vi "Seatingchart.vi"(5 "selected seats before":i32[](array[numeric])) -> (0 "No seat":bool, 1 "selected seats after":i32[](array[numeric]), 2 "seats selected by user":i32[](array[numeric]), 3 "No. of seats choosen":i32, 4 "Cancel":bool)   [LabVIEW 2014]
panel:
  out "No. of seats want to choose":i32
  out "th seat you choose":i32
  out "index":i32
  in  "Seating chart":T1
  in  "stop":bool
  # "1"
  # "2"
  # "3"
  # "4"
  # "5"
  # "6"
  # "A"
  # "A"
  # "B"
  # "B"
  # "C"
  # "C"
  # "D"
  # "D"
  # "E"
  # "E"
  # "F"
  # "F"
  # "G"
  # "G"
  # "H"
  # "H"
  # "1"
  # "2"
  # "3"
  # "4"
  # "5"
  # "6"
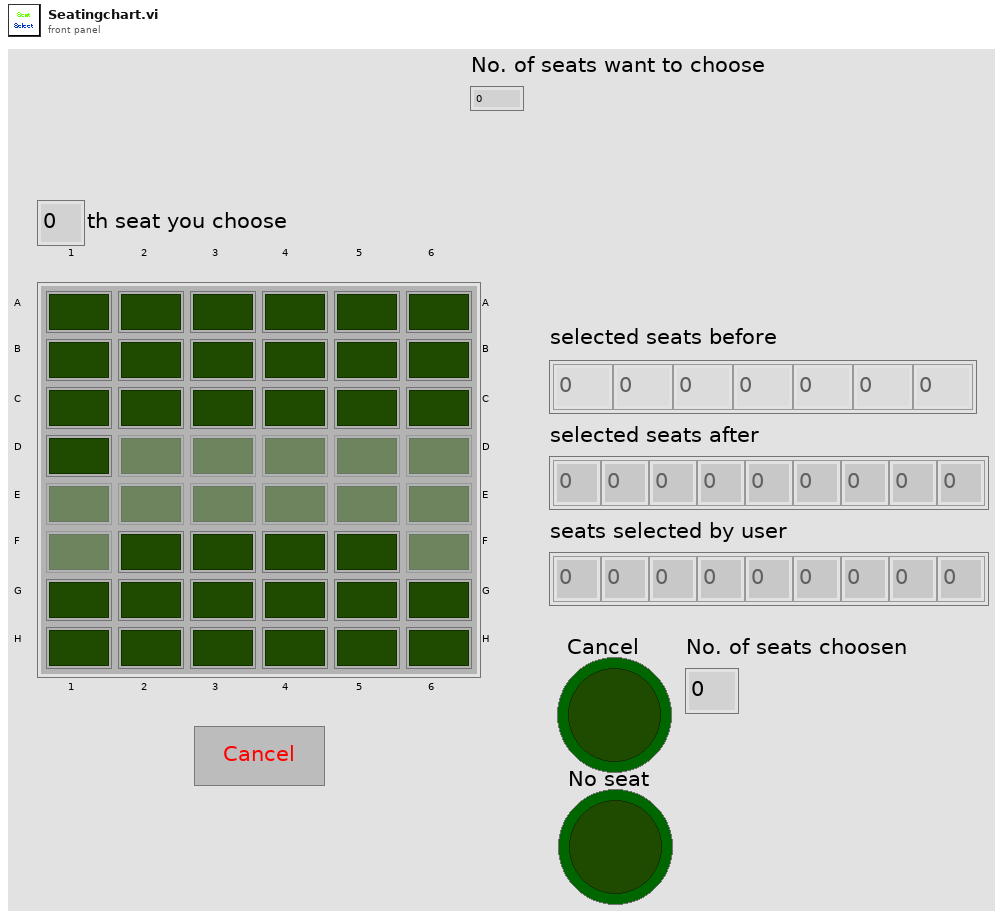
[diagram p1: front panel]
types:
  T1 = cluster{"Boolean":bool, "Boolean 2":bool, "Boolean 3":bool, "Boolean 4":bool, "Boolean 5":bool, "Boolean 6":bool, "Boolean 7":bool, "Boolean 8":bool, "Boolean 9":bool, "Boolean 10":bool, "Boolean 11":bool, "Boolean 12":bool, "Boolean 13":bool, "Boolean 14":bool, "Boolean 15":bool, "Boolean 16":bool, "Boolean 17":bool, "Boolean 18":bool, "Boolean 19":bool, "Boolean 20":bool, "Boolean 21":bool, "Boolean 22":bool, "Boolean 23":bool, "Boolean 24":bool, "Boolean 25":bool, "Boolean 26":bool, "Boolean 27":bool, "Boolean 28":bool, "Boolean 29":bool, "Boolean 30":bool, "Boolean 31":bool, "Boolean 32":bool, "Boolean 33":bool, "Boolean 34":bool, "Boolean 35":bool, "Boolean 36":bool, "Boolean 37":bool, "Boolean 38":bool, "Boolean 39":bool, "Boolean 40":bool, "Boolean 41":bool, "Boolean 42":bool, "Boolean 43":bool, "Boolean 44":bool, "Boolean 45":bool, "Boolean 46":bool, "Boolean 47":bool, "Boolean 48":bool}
  T2 = enum8{"Enabled", "Disabled", "Disabled and Grayed Out"}
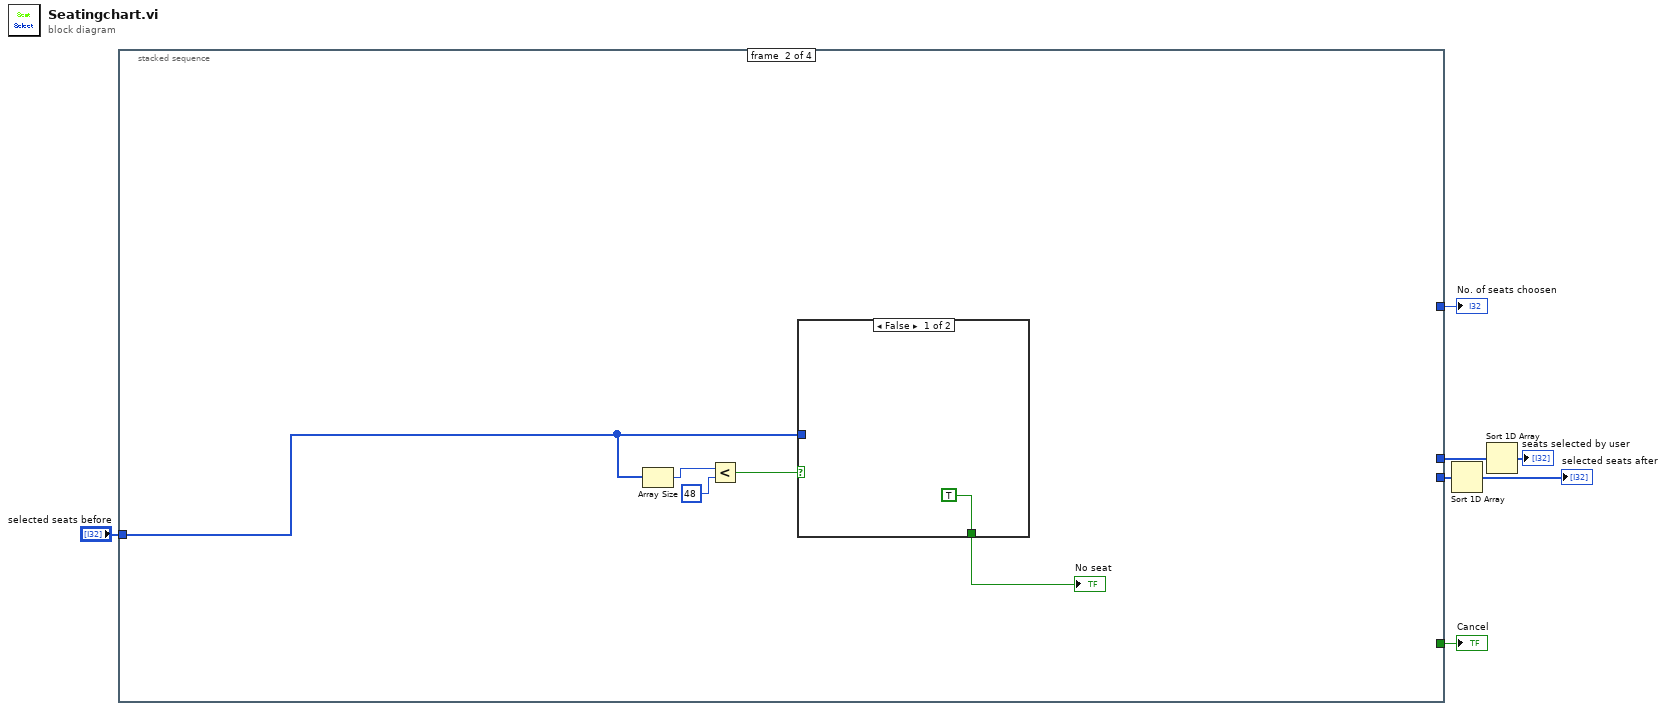
[diagram p0: block diagram]
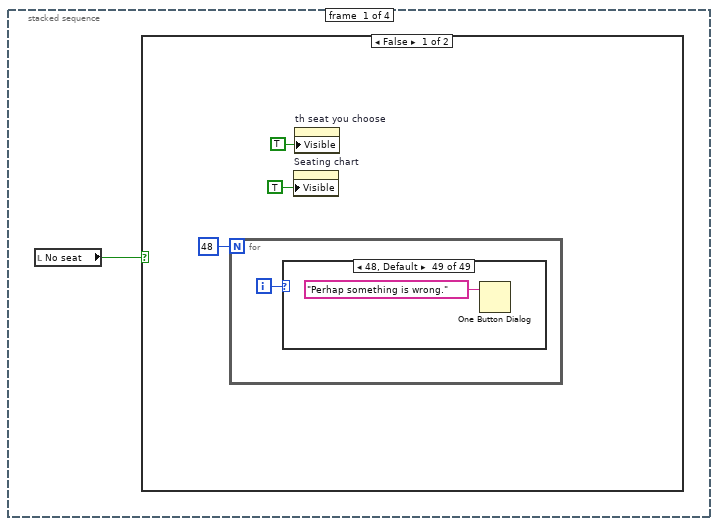
[diagram p2: hidden frame]
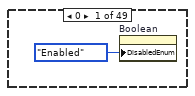
[diagram p3: hidden frame]
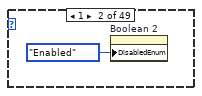
[diagram p4: hidden frame]
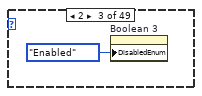
[diagram p5: hidden frame]
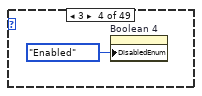
[diagram p6: hidden frame]
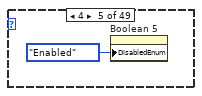
[diagram p7: hidden frame]
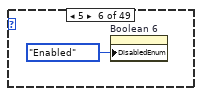
[diagram p8: hidden frame]
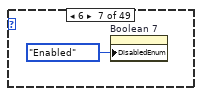
[diagram p9: hidden frame]
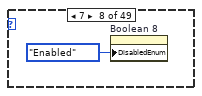
[diagram p10: hidden frame]
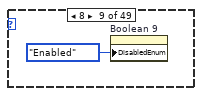
[diagram p11: hidden frame]
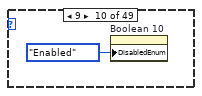
[diagram p12: hidden frame]
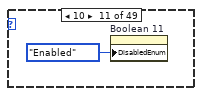
[diagram p13: hidden frame]
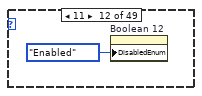
[diagram p14: hidden frame]
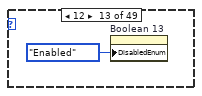
[diagram p15: hidden frame]
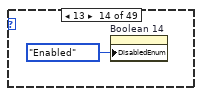
[diagram p16: hidden frame]
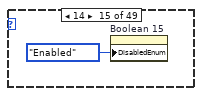
[diagram p17: hidden frame]
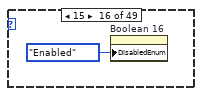
[diagram p18: hidden frame]
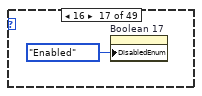
[diagram p19: hidden frame]
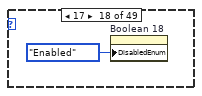
[diagram p20: hidden frame]
diagram:
  n1 = stacked-sequence {
    tunnel: [_ _ _ w130] -> w6
    tunnel: [_ _ _ w128] -> w7
    tunnel: "selected seats before" -> [_ w66 w72 w129]
    tunnel: [_ _ _ w127] -> w4
    tunnel: [_ _ _ w126] -> w3
    frame #0 {
      n2 = local read "No seat"() -> (w8:bool)
      n3 = case shown="False" w8 {
        frame False {
          n4 = for {
            N: 48 -> [_]
            i -> [w12]
            n5 = case shown="48, Default" w12 {
              frame 0 {
                n6 = property on="Boolean" class="Bool"("DisabledEnum"=T2."Enabled" ("Disabled")) -> ()  [unwired: 2 in, 2 out]
              }
              frame 1 {
                n7 = property on="Boolean 2" class="Bool"("DisabledEnum"=T2."Enabled" ("Disabled")) -> ()  [unwired: 2 in, 2 out]
              }
              frame 2 {
                n8 = property on="Boolean 3" class="Bool"("DisabledEnum"=T2."Enabled" ("Disabled")) -> ()  [unwired: 2 in, 2 out]
              }
              frame 3 {
                n9 = property on="Boolean 4" class="Bool"("DisabledEnum"=T2."Enabled" ("Disabled")) -> ()  [unwired: 2 in, 2 out]
              }
              frame 4 {
                n10 = property on="Boolean 5" class="Bool"("DisabledEnum"=T2."Enabled" ("Disabled")) -> ()  [unwired: 2 in, 2 out]
              }
              frame 5 {
                n11 = property on="Boolean 6" class="Bool"("DisabledEnum"=T2."Enabled" ("Disabled")) -> ()  [unwired: 2 in, 2 out]
              }
              frame 6 {
                n12 = property on="Boolean 7" class="Bool"("DisabledEnum"=T2."Enabled" ("Disabled")) -> ()  [unwired: 2 in, 2 out]
              }
              frame 7 {
                n13 = property on="Boolean 8" class="Bool"("DisabledEnum"=T2."Enabled" ("Disabled")) -> ()  [unwired: 2 in, 2 out]
              }
              frame 8 {
                n14 = property on="Boolean 9" class="Bool"("DisabledEnum"=T2."Enabled" ("Disabled")) -> ()  [unwired: 2 in, 2 out]
              }
              frame 9 {
                n15 = property on="Boolean 10" class="Bool"("DisabledEnum"=T2."Enabled" ("Disabled")) -> ()  [unwired: 2 in, 2 out]
              }
              frame 10 {
                n16 = property on="Boolean 11" class="Bool"("DisabledEnum"=T2."Enabled" ("Disabled")) -> ()  [unwired: 2 in, 2 out]
              }
              frame 11 {
                n17 = property on="Boolean 12" class="Bool"("DisabledEnum"=T2."Enabled" ("Disabled")) -> ()  [unwired: 2 in, 2 out]
              }
              frame 12 {
                n18 = property on="Boolean 13" class="Bool"("DisabledEnum"=T2."Enabled" ("Disabled")) -> ()  [unwired: 2 in, 2 out]
              }
              frame 13 {
                n19 = property on="Boolean 14" class="Bool"("DisabledEnum"=T2."Enabled" ("Disabled")) -> ()  [unwired: 2 in, 2 out]
              }
              frame 14 {
                n20 = property on="Boolean 15" class="Bool"("DisabledEnum"=T2."Enabled" ("Disabled")) -> ()  [unwired: 2 in, 2 out]
              }
              frame 15 {
                n21 = property on="Boolean 16" class="Bool"("DisabledEnum"=T2."Enabled" ("Disabled")) -> ()  [unwired: 2 in, 2 out]
              }
              frame 16 {
                n22 = property on="Boolean 17" class="Bool"("DisabledEnum"=T2."Enabled" ("Disabled")) -> ()  [unwired: 2 in, 2 out]
              }
              frame 17 {
                n23 = property on="Boolean 18" class="Bool"("DisabledEnum"=T2."Enabled" ("Disabled")) -> ()  [unwired: 2 in, 2 out]
              }
              frame 18 {
                n24 = property on="Boolean 19" class="Bool"("DisabledEnum"=T2."Enabled" ("Disabled")) -> ()  [unwired: 2 in, 2 out]
              }
              frame 19 {
                n25 = property on="Boolean 20" class="Bool"("DisabledEnum"=T2."Enabled" ("Disabled")) -> ()  [unwired: 2 in, 2 out]
              }
              frame 20 {
                n26 = property on="Boolean 21" class="Bool"("DisabledEnum"=T2."Enabled" ("Disabled")) -> ()  [unwired: 2 in, 2 out]
              }
              frame 21 {
                n27 = property on="Boolean 22" class="Bool"("DisabledEnum"=T2."Enabled" ("Disabled")) -> ()  [unwired: 2 in, 2 out]
              }
              frame 22 {
                n28 = property on="Boolean 23" class="Bool"("DisabledEnum"=T2."Enabled" ("Disabled")) -> ()  [unwired: 2 in, 2 out]
              }
              frame 23 {
                n29 = property on="Boolean 24" class="Bool"("DisabledEnum"=T2."Enabled" ("Disabled")) -> ()  [unwired: 2 in, 2 out]
              }
              frame 24 {
                n30 = property on="Boolean 25" class="Bool"("DisabledEnum"=T2."Enabled" ("Disabled")) -> ()  [unwired: 2 in, 2 out]
              }
              frame 25 {
                n31 = property on="Boolean 26" class="Bool"("DisabledEnum"=T2."Enabled" ("Disabled")) -> ()  [unwired: 2 in, 2 out]
              }
              frame 26 {
                n32 = property on="Boolean 27" class="Bool"("DisabledEnum"=T2."Enabled" ("Disabled")) -> ()  [unwired: 2 in, 2 out]
              }
              frame 27 {
                n33 = property on="Boolean 28" class="Bool"("DisabledEnum"=T2."Enabled" ("Disabled")) -> ()  [unwired: 2 in, 2 out]
              }
              frame 28 {
                n34 = property on="Boolean 29" class="Bool"("DisabledEnum"=T2."Enabled" ("Disabled")) -> ()  [unwired: 2 in, 2 out]
              }
              frame 29 {
                n35 = property on="Boolean 30" class="Bool"("DisabledEnum"=T2."Enabled" ("Disabled")) -> ()  [unwired: 2 in, 2 out]
              }
              frame 30 {
                n36 = property on="Boolean 31" class="Bool"("DisabledEnum"=T2."Enabled" ("Disabled")) -> ()  [unwired: 2 in, 2 out]
              }
              frame 31 {
                n37 = property on="Boolean 32" class="Bool"("DisabledEnum"=T2."Enabled" ("Disabled")) -> ()  [unwired: 2 in, 2 out]
              }
              frame 32 {
                n38 = property on="Boolean 33" class="Bool"("DisabledEnum"=T2."Enabled" ("Disabled")) -> ()  [unwired: 2 in, 2 out]
              }
              frame 33 {
                n39 = property on="Boolean 34" class="Bool"("DisabledEnum"=T2."Enabled" ("Disabled")) -> ()  [unwired: 2 in, 2 out]
              }
              frame 34 {
                n40 = property on="Boolean 35" class="Bool"("DisabledEnum"=T2."Enabled" ("Disabled")) -> ()  [unwired: 2 in, 2 out]
              }
              frame 35 {
                n41 = property on="Boolean 36" class="Bool"("DisabledEnum"=T2."Enabled" ("Disabled")) -> ()  [unwired: 2 in, 2 out]
              }
              frame 36 {
                n42 = property on="Boolean 37" class="Bool"("DisabledEnum"=T2."Enabled" ("Disabled")) -> ()  [unwired: 2 in, 2 out]
              }
              frame 37 {
                n43 = property on="Boolean 38" class="Bool"("DisabledEnum"=T2."Enabled" ("Disabled")) -> ()  [unwired: 2 in, 2 out]
              }
              frame 38 {
                n44 = property on="Boolean 39" class="Bool"("DisabledEnum"=T2."Enabled" ("Disabled")) -> ()  [unwired: 2 in, 2 out]
              }
              frame 39 {
                n45 = property on="Boolean 40" class="Bool"("DisabledEnum"=T2."Enabled" ("Disabled")) -> ()  [unwired: 2 in, 2 out]
              }
              frame 40 {
                n46 = property on="Boolean 41" class="Bool"("DisabledEnum"=T2."Enabled" ("Disabled")) -> ()  [unwired: 2 in, 2 out]
              }
              frame 41 {
                n47 = property on="Boolean 42" class="Bool"("DisabledEnum"=T2."Enabled" ("Disabled")) -> ()  [unwired: 2 in, 2 out]
              }
              frame 42 {
                n48 = property on="Boolean 43" class="Bool"("DisabledEnum"=T2."Enabled" ("Disabled")) -> ()  [unwired: 2 in, 2 out]
              }
              frame 43 {
                n49 = property on="Boolean 44" class="Bool"("DisabledEnum"=T2."Enabled" ("Disabled")) -> ()  [unwired: 2 in, 2 out]
              }
              frame 44 {
                n50 = property on="Boolean 45" class="Bool"("DisabledEnum"=T2."Enabled" ("Disabled")) -> ()  [unwired: 2 in, 2 out]
              }
              frame 45 {
                n51 = property on="Boolean 46" class="Bool"("DisabledEnum"=T2."Enabled" ("Disabled")) -> ()  [unwired: 2 in, 2 out]
              }
              frame 46 {
                n52 = property on="Boolean 47" class="Bool"("DisabledEnum"=T2."Enabled" ("Disabled")) -> ()  [unwired: 2 in, 2 out]
              }
              frame 47 {
                n53 = property on="Boolean 48" class="Bool"("DisabledEnum"=T2."Enabled" ("Disabled")) -> ()  [unwired: 2 in, 2 out]
              }
              frame 48, Default {
                n54 = One Button Dialog(message="Perhap something is wrong.") -> ()  [unwired: 1 in, 1 out]
              }
            }
          }
          n55 = property on="Seating chart" class="Clust"("Visible"=TRUE) -> ()  [unwired: 2 in, 2 out]
          n56 = property on="th seat you choose" class="DigNum (strict)"("Visible"=TRUE) -> ()  [unwired: 2 in, 2 out]
        }
        frame True {
        }
      }
    }
    frame #1 {
      n57 = Array Size(array=w66) -> (size(s)=w62:i32)
      n58 = Less?(x=w62, y=48 ("x")) -> (x < y?=w65:bool)
      n59 = case shown="False" w65 {
        tunnel: w66 -> [_ w70]
        tunnel: [TRUE FALSE] -> w64
        frame False {
        }
        frame True {
          n60 = call "how_many_seats.vi"("selected seats before"=w70) -> ("How many seats do \nyou want to choose?\n(O)"=→"No. of seats want to choose":i32)
        }
      }
      "No seat" <- w64
    }
    frame #2 {
      n61 = local read "No seat"() -> (w71:bool)
      n62 = case shown="False" w71 {
        tunnel: w72 -> [w73 _]
        frame False {
          n63 = Array Size(array=w73) -> (size(s)=w74:i32)
          n64 = for {
            N: w74 -> [_]
            tunnel: w73 -> [w75] mode=indexing
            n65 = case shown="48, Default" w75 {
              frame 0 {
                n66 = property on="Boolean" class="Bool"("DisabledEnum"=T2."Disabled and Grayed Out" ("Disabled")) -> ()  [unwired: 2 in, 2 out]
              }
              frame 1 {
                n67 = property on="Boolean 2" class="Bool"("DisabledEnum"=T2."Disabled and Grayed Out" ("Disabled")) -> ()  [unwired: 2 in, 2 out]
              }
              frame 2 {
                n68 = property on="Boolean 3" class="Bool"("DisabledEnum"=T2."Disabled and Grayed Out" ("Disabled")) -> ()  [unwired: 2 in, 2 out]
              }
              frame 3 {
                n69 = property on="Boolean 4" class="Bool"("DisabledEnum"=T2."Disabled and Grayed Out" ("Disabled")) -> ()  [unwired: 2 in, 2 out]
              }
              frame 4 {
                n70 = property on="Boolean 5" class="Bool"("DisabledEnum"=T2."Disabled and Grayed Out" ("Disabled")) -> ()  [unwired: 2 in, 2 out]
              }
              frame 5 {
                n71 = property on="Boolean 6" class="Bool"("DisabledEnum"=T2."Disabled and Grayed Out" ("Disabled")) -> ()  [unwired: 2 in, 2 out]
              }
              frame 6 {
                n72 = property on="Boolean 7" class="Bool"("DisabledEnum"=T2."Disabled and Grayed Out" ("Disabled")) -> ()  [unwired: 2 in, 2 out]
              }
              frame 7 {
                n73 = property on="Boolean 8" class="Bool"("DisabledEnum"=T2."Disabled and Grayed Out" ("Disabled")) -> ()  [unwired: 2 in, 2 out]
              }
              frame 8 {
                n74 = property on="Boolean 9" class="Bool"("DisabledEnum"=T2."Disabled and Grayed Out" ("Disabled")) -> ()  [unwired: 2 in, 2 out]
              }
              frame 9 {
                n75 = property on="Boolean 10" class="Bool"("DisabledEnum"=T2."Disabled and Grayed Out" ("Disabled")) -> ()  [unwired: 2 in, 2 out]
              }
              frame 10 {
                n76 = property on="Boolean 11" class="Bool"("DisabledEnum"=T2."Disabled and Grayed Out" ("Disabled")) -> ()  [unwired: 2 in, 2 out]
              }
              frame 11 {
                n77 = property on="Boolean 12" class="Bool"("DisabledEnum"=T2."Disabled and Grayed Out" ("Disabled")) -> ()  [unwired: 2 in, 2 out]
              }
              frame 12 {
                n78 = property on="Boolean 13" class="Bool"("DisabledEnum"=T2."Disabled and Grayed Out" ("Disabled")) -> ()  [unwired: 2 in, 2 out]
              }
              frame 13 {
                n79 = property on="Boolean 14" class="Bool"("DisabledEnum"=T2."Disabled and Grayed Out" ("Disabled")) -> ()  [unwired: 2 in, 2 out]
              }
              frame 14 {
                n80 = property on="Boolean 15" class="Bool"("DisabledEnum"=T2."Disabled and Grayed Out" ("Disabled")) -> ()  [unwired: 2 in, 2 out]
              }
              frame 15 {
                n81 = property on="Boolean 16" class="Bool"("DisabledEnum"=T2."Disabled and Grayed Out" ("Disabled")) -> ()  [unwired: 2 in, 2 out]
              }
              frame 16 {
                n82 = property on="Boolean 17" class="Bool"("DisabledEnum"=T2."Disabled and Grayed Out" ("Disabled")) -> ()  [unwired: 2 in, 2 out]
              }
              frame 17 {
                n83 = property on="Boolean 18" class="Bool"("DisabledEnum"=T2."Disabled and Grayed Out" ("Disabled")) -> ()  [unwired: 2 in, 2 out]
              }
              frame 18 {
                n84 = property on="Boolean 19" class="Bool"("DisabledEnum"=T2."Disabled and Grayed Out" ("Disabled")) -> ()  [unwired: 2 in, 2 out]
              }
              frame 19 {
                n85 = property on="Boolean 20" class="Bool"("DisabledEnum"=T2."Disabled and Grayed Out" ("Disabled")) -> ()  [unwired: 2 in, 2 out]
              }
              frame 20 {
                n86 = property on="Boolean 21" class="Bool"("DisabledEnum"=T2."Disabled and Grayed Out" ("Disabled")) -> ()  [unwired: 2 in, 2 out]
              }
              frame 21 {
                n87 = property on="Boolean 22" class="Bool"("DisabledEnum"=T2."Disabled and Grayed Out" ("Disabled")) -> ()  [unwired: 2 in, 2 out]
              }
              frame 22 {
                n88 = property on="Boolean 23" class="Bool"("DisabledEnum"=T2."Disabled and Grayed Out" ("Disabled")) -> ()  [unwired: 2 in, 2 out]
              }
              frame 23 {
                n89 = property on="Boolean 24" class="Bool"("DisabledEnum"=T2."Disabled and Grayed Out" ("Disabled")) -> ()  [unwired: 2 in, 2 out]
              }
              frame 24 {
                n90 = property on="Boolean 25" class="Bool"("DisabledEnum"=T2."Disabled and Grayed Out" ("Disabled")) -> ()  [unwired: 2 in, 2 out]
              }
              frame 25 {
                n91 = property on="Boolean 26" class="Bool"("DisabledEnum"=T2."Disabled and Grayed Out" ("Disabled")) -> ()  [unwired: 2 in, 2 out]
              }
              frame 26 {
                n92 = property on="Boolean 27" class="Bool"("DisabledEnum"=T2."Disabled and Grayed Out" ("Disabled")) -> ()  [unwired: 2 in, 2 out]
              }
              frame 27 {
                n93 = property on="Boolean 28" class="Bool"("DisabledEnum"=T2."Disabled and Grayed Out" ("Disabled")) -> ()  [unwired: 2 in, 2 out]
              }
              frame 28 {
                n94 = property on="Boolean 29" class="Bool"("DisabledEnum"=T2."Disabled and Grayed Out" ("Disabled")) -> ()  [unwired: 2 in, 2 out]
              }
              frame 29 {
                n95 = property on="Boolean 30" class="Bool"("DisabledEnum"=T2."Disabled and Grayed Out" ("Disabled")) -> ()  [unwired: 2 in, 2 out]
              }
              frame 30 {
                n96 = property on="Boolean 31" class="Bool"("DisabledEnum"=T2."Disabled and Grayed Out" ("Disabled")) -> ()  [unwired: 2 in, 2 out]
              }
              frame 31 {
                n97 = property on="Boolean 32" class="Bool"("DisabledEnum"=T2."Disabled and Grayed Out" ("Disabled")) -> ()  [unwired: 2 in, 2 out]
              }
              frame 32 {
                n98 = property on="Boolean 33" class="Bool"("DisabledEnum"=T2."Disabled and Grayed Out" ("Disabled")) -> ()  [unwired: 2 in, 2 out]
              }
              frame 33 {
                n99 = property on="Boolean 34" class="Bool"("DisabledEnum"=T2."Disabled and Grayed Out" ("Disabled")) -> ()  [unwired: 2 in, 2 out]
              }
              frame 34 {
                n100 = property on="Boolean 35" class="Bool"("DisabledEnum"=T2."Disabled and Grayed Out" ("Disabled")) -> ()  [unwired: 2 in, 2 out]
              }
              frame 35 {
                n101 = property on="Boolean 36" class="Bool"("DisabledEnum"=T2."Disabled and Grayed Out" ("Disabled")) -> ()  [unwired: 2 in, 2 out]
              }
              frame 36 {
                n102 = property on="Boolean 37" class="Bool"("DisabledEnum"=T2."Disabled and Grayed Out" ("Disabled")) -> ()  [unwired: 2 in, 2 out]
              }
              frame 37 {
                n103 = property on="Boolean 38" class="Bool"("DisabledEnum"=T2."Disabled and Grayed Out" ("Disabled")) -> ()  [unwired: 2 in, 2 out]
              }
              frame 38 {
                n104 = property on="Boolean 39" class="Bool"("DisabledEnum"=T2."Disabled and Grayed Out" ("Disabled")) -> ()  [unwired: 2 in, 2 out]
              }
              frame 39 {
                n105 = property on="Boolean 40" class="Bool"("DisabledEnum"=T2."Disabled and Grayed Out" ("Disabled")) -> ()  [unwired: 2 in, 2 out]
              }
              frame 40 {
                n106 = property on="Boolean 41" class="Bool"("DisabledEnum"=T2."Disabled and Grayed Out" ("Disabled")) -> ()  [unwired: 2 in, 2 out]
              }
              frame 41 {
                n107 = property on="Boolean 42" class="Bool"("DisabledEnum"=T2."Disabled and Grayed Out" ("Disabled")) -> ()  [unwired: 2 in, 2 out]
              }
              frame 42 {
                n108 = property on="Boolean 43" class="Bool"("DisabledEnum"=T2."Disabled and Grayed Out" ("Disabled")) -> ()  [unwired: 2 in, 2 out]
              }
              frame 43 {
                n109 = property on="Boolean 44" class="Bool"("DisabledEnum"=T2."Disabled and Grayed Out" ("Disabled")) -> ()  [unwired: 2 in, 2 out]
              }
              frame 44 {
                n110 = property on="Boolean 45" class="Bool"("DisabledEnum"=T2."Disabled and Grayed Out" ("Disabled")) -> ()  [unwired: 2 in, 2 out]
              }
              frame 45 {
                n111 = property on="Boolean 46" class="Bool"("DisabledEnum"=T2."Disabled and Grayed Out" ("Disabled")) -> ()  [unwired: 2 in, 2 out]
              }
              frame 46 {
                n112 = property on="Boolean 47" class="Bool"("DisabledEnum"=T2."Disabled and Grayed Out" ("Disabled")) -> ()  [unwired: 2 in, 2 out]
              }
              frame 47 {
                n113 = property on="Boolean 48" class="Bool"("DisabledEnum"=T2."Disabled and Grayed Out" ("Disabled")) -> ()  [unwired: 2 in, 2 out]
              }
              frame 48, Default {
                n114 = One Button Dialog(message="Perhap something is wrong.") -> ()  [unwired: 1 in, 1 out]
              }
            }
          }
        }
        frame True {
        }
      }
    }
    frame #3 {
      n115 = local read "No seat"() -> (w125:bool)
      n116 = case shown="True" w125 {
        tunnel: [w138 w836] -> w130
        tunnel: w129 -> [w136 _]
        tunnel: [w135 w836] -> w128
        tunnel: [w134 FALSE ("stop")] -> w127
        tunnel: [w132 0 ("No. of seats want to choose")] -> w126
        frame False {
          n117 = local read "No. of seats want to choose"() -> (w133:i32)
          n118 = while {
            shift-right: [w151] -> _
            shift-left: w133 -> [w150]
            shift-right: [w156] -> w137
            shift-left: i32[] [] ("Array") -> [w157]
            tunnel: ["stop"] -> w134
            tunnel: w133 -> [w147]
            tunnel: [w147] -> w131
            stop <- w154 stop-if-true
            n119 = Cluster To Array(cluster="Seating chart") -> (array=w158:bool[])
            n120 = Search 1D Array(1D array=w158, element=TRUE) -> (index of element=w155:i32)  [unwired: 1 in]
            "index" <- w155
            n121 = case shown="47" w155 {
              selector: w155 -> [w161 w175 w189 w203 w217 w231 w245 w259 w273 w287 w301 w315 w329 w343 w357 w371 w385 w399 w413 w427 w441 w455 w469 w483 w497 w511 w525 w539 w553 w567 w581 w595 w609 w623 w637 w651 w665 w679 w693 w707 w721 w735 w749 w763 w777 w791 w805 w819 _]
              tunnel: w150 -> [w165 w179 w193 w207 w221 w235 w249 w263 w277 w291 w305 w319 w333 w347 w361 w375 w389 w403 w417 w431 w445 w459 w473 w487 w501 w515 w529 w543 w557 w571 w585 w599 w613 w627 w641 w655 w669 w683 w697 w711 w725 w739 w753 w767 w781 w795 w809 w823 w834]
              tunnel: [w164 w178 w192 w206 w220 w234 w248 w262 w276 w290 w304 w318 w332 w346 w360 w374 w388 w402 w416 w430 w444 w458 w472 w486 w500 w514 w528 w542 w556 w570 w584 w598 w612 w626 w640 w654 w668 w682 w696 w710 w724 w738 w752 w766 w780 w794 w808 w822 w834] -> w151
              tunnel: w157 -> [w163 w177 w191 w205 w219 w233 w247 w261 w275 w289 w303 w317 w331 w345 w359 w373 w387 w401 w415 w429 w443 w457 w471 w485 w499 w513 w527 w541 w555 w569 w583 w597 w611 w625 w639 w653 w667 w681 w695 w709 w723 w737 w751 w765 w779 w793 w807 w821 w833]
              tunnel: [w162 w176 w190 w204 w218 w232 w246 w260 w274 w288 w302 w316 w330 w344 w358 w372 w386 w400 w414 w428 w442 w456 w470 w484 w498 w512 w526 w540 w554 w568 w582 w596 w610 w624 w638 w652 w666 w680 w694 w708 w722 w736 w750 w764 w778 w792 w806 w820 w833] -> w156
              frame 0 {
                n122 = call "select_seat_comfirm.vi"("choose index"=w161) -> ("Boolean"=w166:bool)
                n123 = case shown="True" w166 {
                  tunnel: w165 -> [w168 w173]
                  tunnel: [w168 w172] -> w164
                  tunnel: w163 -> [w167 w171]
                  tunnel: [w167 w169] -> w162
                  tunnel: w161 -> [_ w170]
                  frame False {
                  }
                  frame True {
                    n124 = Build Array (concatenate)(w171, w170) -> (w169:i32[])
                    n125 = Decrement(x=w173) -> (x-1=w172:i32)
                    n126 = property on="Boolean" class="Bool"("DisabledEnum"=T2."Disabled and Grayed Out" ("Disabled")) -> ()  [unwired: 2 in, 2 out]
                  }
                }
              }
              frame 1 {
                n127 = call "select_seat_comfirm.vi"("choose index"=w175) -> ("Boolean"=w180:bool)
                n128 = case shown="True" w180 {
                  tunnel: w179 -> [w182 w188]
                  tunnel: [w182 w187] -> w178
                  tunnel: w177 -> [w181 w186]
                  tunnel: [w181 w184] -> w176
                  tunnel: w175 -> [_ w185]
                  frame False {
                  }
                  frame True {
                    n129 = Build Array (concatenate)(w186, w185) -> (w184:i32[])
                    n130 = Decrement(x=w188) -> (x-1=w187:i32)
                    n131 = property on="Boolean 2" class="Bool"("DisabledEnum"=T2."Disabled and Grayed Out" ("Disabled")) -> ()  [unwired: 2 in, 2 out]
                  }
                }
              }
              frame 2 {
                n132 = call "select_seat_comfirm.vi"("choose index"=w189) -> ("Boolean"=w194:bool)
                n133 = case shown="True" w194 {
                  tunnel: w193 -> [w196 w202]
                  tunnel: [w196 w201] -> w192
                  tunnel: w191 -> [w195 w200]
                  tunnel: [w195 w198] -> w190
                  tunnel: w189 -> [_ w199]
                  frame False {
                  }
                  frame True {
                    n134 = Build Array (concatenate)(w200, w199) -> (w198:i32[])
                    n135 = Decrement(x=w202) -> (x-1=w201:i32)
                    n136 = property on="Boolean 3" class="Bool"("DisabledEnum"=T2."Disabled and Grayed Out" ("Disabled")) -> ()  [unwired: 2 in, 2 out]
                  }
                }
              }
              frame 3 {
                n137 = call "select_seat_comfirm.vi"("choose index"=w203) -> ("Boolean"=w208:bool)
                n138 = case shown="True" w208 {
                  tunnel: w207 -> [w210 w216]
                  tunnel: [w210 w215] -> w206
                  tunnel: w205 -> [w209 w214]
                  tunnel: [w209 w212] -> w204
                  tunnel: w203 -> [_ w213]
                  frame False {
                  }
                  frame True {
                    n139 = Build Array (concatenate)(w214, w213) -> (w212:i32[])
                    n140 = Decrement(x=w216) -> (x-1=w215:i32)
                    n141 = property on="Boolean 4" class="Bool"("DisabledEnum"=T2."Disabled and Grayed Out" ("Disabled")) -> ()  [unwired: 2 in, 2 out]
                  }
                }
              }
              frame 4 {
                n142 = call "select_seat_comfirm.vi"("choose index"=w217) -> ("Boolean"=w222:bool)
                n143 = case shown="True" w222 {
                  tunnel: w221 -> [w224 w230]
                  tunnel: [w224 w229] -> w220
                  tunnel: w219 -> [w223 w228]
                  tunnel: [w223 w226] -> w218
                  tunnel: w217 -> [_ w227]
                  frame False {
                  }
                  frame True {
                    n144 = Build Array (concatenate)(w228, w227) -> (w226:i32[])
                    n145 = Decrement(x=w230) -> (x-1=w229:i32)
                    n146 = property on="Boolean 5" class="Bool"("DisabledEnum"=T2."Disabled and Grayed Out" ("Disabled")) -> ()  [unwired: 2 in, 2 out]
                  }
                }
              }
              frame 5 {
                n147 = call "select_seat_comfirm.vi"("choose index"=w231) -> ("Boolean"=w236:bool)
                n148 = case shown="True" w236 {
                  tunnel: w235 -> [w238 w244]
                  tunnel: [w238 w243] -> w234
                  tunnel: w233 -> [w237 w242]
                  tunnel: [w237 w240] -> w232
                  tunnel: w231 -> [_ w241]
                  frame False {
                  }
                  frame True {
                    n149 = Build Array (concatenate)(w242, w241) -> (w240:i32[])
                    n150 = Decrement(x=w244) -> (x-1=w243:i32)
                    n151 = property on="Boolean 6" class="Bool"("DisabledEnum"=T2."Disabled and Grayed Out" ("Disabled")) -> ()  [unwired: 2 in, 2 out]
                  }
                }
              }
              frame 6 {
                n152 = call "select_seat_comfirm.vi"("choose index"=w245) -> ("Boolean"=w250:bool)
                n153 = case shown="True" w250 {
                  tunnel: w249 -> [w252 w258]
                  tunnel: [w252 w257] -> w248
                  tunnel: w247 -> [w251 w256]
                  tunnel: [w251 w254] -> w246
                  tunnel: w245 -> [_ w255]
                  frame False {
                  }
                  frame True {
                    n154 = Build Array (concatenate)(w256, w255) -> (w254:i32[])
                    n155 = Decrement(x=w258) -> (x-1=w257:i32)
                    n156 = property on="Boolean 7" class="Bool"("DisabledEnum"=T2."Disabled and Grayed Out" ("Disabled")) -> ()  [unwired: 2 in, 2 out]
                  }
                }
              }
              frame 7 {
                n157 = call "select_seat_comfirm.vi"("choose index"=w259) -> ("Boolean"=w264:bool)
                n158 = case shown="True" w264 {
                  tunnel: w263 -> [w266 w272]
                  tunnel: [w266 w271] -> w262
                  tunnel: w261 -> [w265 w270]
                  tunnel: [w265 w268] -> w260
                  tunnel: w259 -> [_ w269]
                  frame False {
                  }
                  frame True {
                    n159 = Build Array (concatenate)(w270, w269) -> (w268:i32[])
                    n160 = Decrement(x=w272) -> (x-1=w271:i32)
                    n161 = property on="Boolean 8" class="Bool"("DisabledEnum"=T2."Disabled and Grayed Out" ("Disabled")) -> ()  [unwired: 2 in, 2 out]
                  }
                }
              }
              frame 8 {
                n162 = call "select_seat_comfirm.vi"("choose index"=w273) -> ("Boolean"=w278:bool)
                n163 = case shown="True" w278 {
                  tunnel: w277 -> [w280 w286]
                  tunnel: [w280 w285] -> w276
                  tunnel: w275 -> [w279 w284]
                  tunnel: [w279 w282] -> w274
                  tunnel: w273 -> [_ w283]
                  frame False {
                  }
                  frame True {
                    n164 = Build Array (concatenate)(w284, w283) -> (w282:i32[])
                    n165 = Decrement(x=w286) -> (x-1=w285:i32)
                    n166 = property on="Boolean 9" class="Bool"("DisabledEnum"=T2."Disabled and Grayed Out" ("Disabled")) -> ()  [unwired: 2 in, 2 out]
                  }
                }
              }
              frame 9 {
                n167 = call "select_seat_comfirm.vi"("choose index"=w287) -> ("Boolean"=w292:bool)
                n168 = case shown="True" w292 {
                  tunnel: w291 -> [w294 w300]
                  tunnel: [w294 w299] -> w290
                  tunnel: w289 -> [w293 w298]
                  tunnel: [w293 w296] -> w288
                  tunnel: w287 -> [_ w297]
                  frame False {
                  }
                  frame True {
                    n169 = Build Array (concatenate)(w298, w297) -> (w296:i32[])
                    n170 = Decrement(x=w300) -> (x-1=w299:i32)
                    n171 = property on="Boolean 10" class="Bool"("DisabledEnum"=T2."Disabled and Grayed Out" ("Disabled")) -> ()  [unwired: 2 in, 2 out]
                  }
                }
              }
              frame 10 {
                n172 = call "select_seat_comfirm.vi"("choose index"=w301) -> ("Boolean"=w306:bool)
                n173 = case shown="True" w306 {
                  tunnel: w305 -> [w308 w314]
                  tunnel: [w308 w313] -> w304
                  tunnel: w303 -> [w307 w312]
                  tunnel: [w307 w310] -> w302
                  tunnel: w301 -> [_ w311]
                  frame False {
                  }
                  frame True {
                    n174 = Build Array (concatenate)(w312, w311) -> (w310:i32[])
                    n175 = Decrement(x=w314) -> (x-1=w313:i32)
                    n176 = property on="Boolean 11" class="Bool"("DisabledEnum"=T2."Disabled and Grayed Out" ("Disabled")) -> ()  [unwired: 2 in, 2 out]
                  }
                }
              }
              frame 11 {
                n177 = call "select_seat_comfirm.vi"("choose index"=w315) -> ("Boolean"=w320:bool)
                n178 = case shown="True" w320 {
                  tunnel: w319 -> [w322 w328]
                  tunnel: [w322 w327] -> w318
                  tunnel: w317 -> [w321 w326]
                  tunnel: [w321 w324] -> w316
                  tunnel: w315 -> [_ w325]
                  frame False {
                  }
                  frame True {
                    n179 = Build Array (concatenate)(w326, w325) -> (w324:i32[])
                    n180 = Decrement(x=w328) -> (x-1=w327:i32)
                    n181 = property on="Boolean 12" class="Bool"("DisabledEnum"=T2."Disabled and Grayed Out" ("Disabled")) -> ()  [unwired: 2 in, 2 out]
                  }
                }
              }
              frame 12 {
                n182 = call "select_seat_comfirm.vi"("choose index"=w329) -> ("Boolean"=w334:bool)
                n183 = case shown="True" w334 {
                  tunnel: w333 -> [w336 w342]
                  tunnel: [w336 w341] -> w332
                  tunnel: w331 -> [w335 w340]
                  tunnel: [w335 w338] -> w330
                  tunnel: w329 -> [_ w339]
                  frame False {
                  }
                  frame True {
                    n184 = Build Array (concatenate)(w340, w339) -> (w338:i32[])
                    n185 = Decrement(x=w342) -> (x-1=w341:i32)
                    n186 = property on="Boolean 13" class="Bool"("DisabledEnum"=T2."Disabled and Grayed Out" ("Disabled")) -> ()  [unwired: 2 in, 2 out]
                  }
                }
              }
              frame 13 {
                n187 = call "select_seat_comfirm.vi"("choose index"=w343) -> ("Boolean"=w348:bool)
                n188 = case shown="True" w348 {
                  tunnel: w347 -> [w350 w356]
                  tunnel: [w350 w355] -> w346
                  tunnel: w345 -> [w349 w354]
                  tunnel: [w349 w352] -> w344
                  tunnel: w343 -> [_ w353]
                  frame False {
                  }
                  frame True {
                    n189 = Build Array (concatenate)(w354, w353) -> (w352:i32[])
                    n190 = Decrement(x=w356) -> (x-1=w355:i32)
                    n191 = property on="Boolean 14" class="Bool"("DisabledEnum"=T2."Disabled and Grayed Out" ("Disabled")) -> ()  [unwired: 2 in, 2 out]
                  }
                }
              }
              frame 14 {
                n192 = call "select_seat_comfirm.vi"("choose index"=w357) -> ("Boolean"=w362:bool)
                n193 = case shown="True" w362 {
                  tunnel: w361 -> [w364 w370]
                  tunnel: [w364 w369] -> w360
                  tunnel: w359 -> [w363 w368]
                  tunnel: [w363 w366] -> w358
                  tunnel: w357 -> [_ w367]
                  frame False {
                  }
                  frame True {
                    n194 = Build Array (concatenate)(w368, w367) -> (w366:i32[])
                    n195 = Decrement(x=w370) -> (x-1=w369:i32)
                    n196 = property on="Boolean 15" class="Bool"("DisabledEnum"=T2."Disabled and Grayed Out" ("Disabled")) -> ()  [unwired: 2 in, 2 out]
                  }
                }
              }
              frame 15 {
                n197 = call "select_seat_comfirm.vi"("choose index"=w371) -> ("Boolean"=w376:bool)
                n198 = case shown="True" w376 {
                  tunnel: w375 -> [w378 w384]
                  tunnel: [w378 w383] -> w374
                  tunnel: w373 -> [w377 w382]
                  tunnel: [w377 w380] -> w372
                  tunnel: w371 -> [_ w381]
                  frame False {
                  }
                  frame True {
                    n199 = Build Array (concatenate)(w382, w381) -> (w380:i32[])
                    n200 = Decrement(x=w384) -> (x-1=w383:i32)
                    n201 = property on="Boolean 16" class="Bool"("DisabledEnum"=T2."Disabled and Grayed Out" ("Disabled")) -> ()  [unwired: 2 in, 2 out]
                  }
                }
              }
              frame 16 {
                n202 = call "select_seat_comfirm.vi"("choose index"=w385) -> ("Boolean"=w390:bool)
                n203 = case shown="True" w390 {
                  tunnel: w389 -> [w392 w398]
                  tunnel: [w392 w397] -> w388
                  tunnel: w387 -> [w391 w396]
                  tunnel: [w391 w394] -> w386
                  tunnel: w385 -> [_ w395]
                  frame False {
                  }
                  frame True {
                    n204 = Build Array (concatenate)(w396, w395) -> (w394:i32[])
                    n205 = Decrement(x=w398) -> (x-1=w397:i32)
                    n206 = property on="Boolean 17" class="Bool"("DisabledEnum"=T2."Disabled and Grayed Out" ("Disabled")) -> ()  [unwired: 2 in, 2 out]
                  }
                }
              }
              frame 17 {
                n207 = call "select_seat_comfirm.vi"("choose index"=w399) -> ("Boolean"=w404:bool)
                n208 = case shown="True" w404 {
                  tunnel: w403 -> [w406 w412]
                  tunnel: [w406 w411] -> w402
                  tunnel: w401 -> [w405 w410]
                  tunnel: [w405 w408] -> w400
                  tunnel: w399 -> [_ w409]
                  frame False {
                  }
                  frame True {
                    n209 = Build Array (concatenate)(w410, w409) -> (w408:i32[])
                    n210 = Decrement(x=w412) -> (x-1=w411:i32)
                    n211 = property on="Boolean 18" class="Bool"("DisabledEnum"=T2."Disabled and Grayed Out" ("Disabled")) -> ()  [unwired: 2 in, 2 out]
                  }
                }
              }
              frame 18 {
                n212 = call "select_seat_comfirm.vi"("choose index"=w413) -> ("Boolean"=w418:bool)
                n213 = case shown="True" w418 {
                  tunnel: w417 -> [w420 w426]
                  tunnel: [w420 w425] -> w416
                  tunnel: w415 -> [w419 w424]
                  tunnel: [w419 w422] -> w414
                  tunnel: w413 -> [_ w423]
                  frame False {
                  }
                  frame True {
                    n214 = Build Array (concatenate)(w424, w423) -> (w422:i32[])
                    n215 = Decrement(x=w426) -> (x-1=w425:i32)
                    n216 = property on="Boolean 19" class="Bool"("DisabledEnum"=T2."Disabled and Grayed Out" ("Disabled")) -> ()  [unwired: 2 in, 2 out]
                  }
                }
              }
              frame 19 {
                n217 = call "select_seat_comfirm.vi"("choose index"=w427) -> ("Boolean"=w432:bool)
                n218 = case shown="True" w432 {
                  tunnel: w431 -> [w434 w440]
                  tunnel: [w434 w439] -> w430
                  tunnel: w429 -> [w433 w438]
                  tunnel: [w433 w436] -> w428
                  tunnel: w427 -> [_ w437]
                  frame False {
                  }
                  frame True {
                    n219 = Build Array (concatenate)(w438, w437) -> (w436:i32[])
                    n220 = Decrement(x=w440) -> (x-1=w439:i32)
                    n221 = property on="Boolean 20" class="Bool"("DisabledEnum"=T2."Disabled and Grayed Out" ("Disabled")) -> ()  [unwired: 2 in, 2 out]
                  }
                }
              }
              frame 20 {
                n222 = call "select_seat_comfirm.vi"("choose index"=w441) -> ("Boolean"=w446:bool)
                n223 = case shown="True" w446 {
                  tunnel: w445 -> [w448 w454]
                  tunnel: [w448 w453] -> w444
                  tunnel: w443 -> [w447 w452]
                  tunnel: [w447 w450] -> w442
                  tunnel: w441 -> [_ w451]
                  frame False {
                  }
                  frame True {
                    n224 = Build Array (concatenate)(w452, w451) -> (w450:i32[])
                    n225 = Decrement(x=w454) -> (x-1=w453:i32)
                    n226 = property on="Boolean 21" class="Bool"("DisabledEnum"=T2."Disabled and Grayed Out" ("Disabled")) -> ()  [unwired: 2 in, 2 out]
                  }
                }
              }
              frame 21 {
                n227 = call "select_seat_comfirm.vi"("choose index"=w455) -> ("Boolean"=w460:bool)
                n228 = case shown="True" w460 {
                  tunnel: w459 -> [w462 w468]
                  tunnel: [w462 w467] -> w458
                  tunnel: w457 -> [w461 w466]
                  tunnel: [w461 w464] -> w456
                  tunnel: w455 -> [_ w465]
                  frame False {
                  }
                  frame True {
                    n229 = Build Array (concatenate)(w466, w465) -> (w464:i32[])
                    n230 = Decrement(x=w468) -> (x-1=w467:i32)
                    n231 = property on="Boolean 22" class="Bool"("DisabledEnum"=T2."Disabled and Grayed Out" ("Disabled")) -> ()  [unwired: 2 in, 2 out]
                  }
                }
              }
              frame 22 {
                n232 = call "select_seat_comfirm.vi"("choose index"=w469) -> ("Boolean"=w474:bool)
                n233 = case shown="True" w474 {
                  tunnel: w473 -> [w476 w482]
                  tunnel: [w476 w481] -> w472
                  tunnel: w471 -> [w475 w480]
                  tunnel: [w475 w478] -> w470
                  tunnel: w469 -> [_ w479]
                  frame False {
                  }
                  frame True {
                    n234 = Build Array (concatenate)(w480, w479) -> (w478:i32[])
                    n235 = Decrement(x=w482) -> (x-1=w481:i32)
                    n236 = property on="Boolean 23" class="Bool"("DisabledEnum"=T2."Disabled and Grayed Out" ("Disabled")) -> ()  [unwired: 2 in, 2 out]
                  }
                }
              }
              frame 23 {
                n237 = call "select_seat_comfirm.vi"("choose index"=w483) -> ("Boolean"=w488:bool)
                n238 = case shown="True" w488 {
                  tunnel: w487 -> [w490 w496]
                  tunnel: [w490 w495] -> w486
                  tunnel: w485 -> [w489 w494]
                  tunnel: [w489 w492] -> w484
                  tunnel: w483 -> [_ w493]
                  frame False {
                  }
                  frame True {
                    n239 = Build Array (concatenate)(w494, w493) -> (w492:i32[])
                    n240 = Decrement(x=w496) -> (x-1=w495:i32)
                    n241 = property on="Boolean 24" class="Bool"("DisabledEnum"=T2."Disabled and Grayed Out" ("Disabled")) -> ()  [unwired: 2 in, 2 out]
                  }
                }
              }
              frame 24 {
                n242 = call "select_seat_comfirm.vi"("choose index"=w497) -> ("Boolean"=w502:bool)
                n243 = case shown="True" w502 {
                  tunnel: w501 -> [w504 w510]
                  tunnel: [w504 w509] -> w500
                  tunnel: w499 -> [w503 w508]
                  tunnel: [w503 w506] -> w498
                  tunnel: w497 -> [_ w507]
                  frame False {
                  }
                  frame True {
                    n244 = Build Array (concatenate)(w508, w507) -> (w506:i32[])
                    n245 = Decrement(x=w510) -> (x-1=w509:i32)
                    n246 = property on="Boolean 25" class="Bool"("DisabledEnum"=T2."Disabled and Grayed Out" ("Disabled")) -> ()  [unwired: 2 in, 2 out]
                  }
                }
              }
              frame 25 {
                n247 = call "select_seat_comfirm.vi"("choose index"=w511) -> ("Boolean"=w516:bool)
                n248 = case shown="True" w516 {
                  tunnel: w515 -> [w518 w524]
                  tunnel: [w518 w523] -> w514
                  tunnel: w513 -> [w517 w522]
                  tunnel: [w517 w520] -> w512
                  tunnel: w511 -> [_ w521]
                  frame False {
                  }
                  frame True {
                    n249 = Build Array (concatenate)(w522, w521) -> (w520:i32[])
                    n250 = Decrement(x=w524) -> (x-1=w523:i32)
                    n251 = property on="Boolean 26" class="Bool"("DisabledEnum"=T2."Disabled and Grayed Out" ("Disabled")) -> ()  [unwired: 2 in, 2 out]
                  }
                }
              }
              frame 26 {
                n252 = call "select_seat_comfirm.vi"("choose index"=w525) -> ("Boolean"=w530:bool)
                n253 = case shown="True" w530 {
                  tunnel: w529 -> [w532 w538]
                  tunnel: [w532 w537] -> w528
                  tunnel: w527 -> [w531 w536]
                  tunnel: [w531 w534] -> w526
                  tunnel: w525 -> [_ w535]
                  frame False {
                  }
                  frame True {
                    n254 = Build Array (concatenate)(w536, w535) -> (w534:i32[])
                    n255 = Decrement(x=w538) -> (x-1=w537:i32)
                    n256 = property on="Boolean 27" class="Bool"("DisabledEnum"=T2."Disabled and Grayed Out" ("Disabled")) -> ()  [unwired: 2 in, 2 out]
                  }
                }
              }
              frame 27 {
                n257 = call "select_seat_comfirm.vi"("choose index"=w539) -> ("Boolean"=w544:bool)
                n258 = case shown="True" w544 {
                  tunnel: w543 -> [w546 w552]
                  tunnel: [w546 w551] -> w542
                  tunnel: w541 -> [w545 w550]
                  tunnel: [w545 w548] -> w540
                  tunnel: w539 -> [_ w549]
                  frame False {
                  }
                  frame True {
                    n259 = Build Array (concatenate)(w550, w549) -> (w548:i32[])
                    n260 = Decrement(x=w552) -> (x-1=w551:i32)
                    n261 = property on="Boolean 28" class="Bool"("DisabledEnum"=T2."Disabled and Grayed Out" ("Disabled")) -> ()  [unwired: 2 in, 2 out]
                  }
                }
              }
              frame 28 {
                n262 = call "select_seat_comfirm.vi"("choose index"=w553) -> ("Boolean"=w558:bool)
                n263 = case shown="True" w558 {
                  tunnel: w557 -> [w560 w566]
                  tunnel: [w560 w565] -> w556
                  tunnel: w555 -> [w559 w564]
                  tunnel: [w559 w562] -> w554
                  tunnel: w553 -> [_ w563]
                  frame False {
                  }
                  frame True {
                    n264 = Build Array (concatenate)(w564, w563) -> (w562:i32[])
                    n265 = Decrement(x=w566) -> (x-1=w565:i32)
                    n266 = property on="Boolean 29" class="Bool"("DisabledEnum"=T2."Disabled and Grayed Out" ("Disabled")) -> ()  [unwired: 2 in, 2 out]
                  }
                }
              }
              frame 29 {
                n267 = call "select_seat_comfirm.vi"("choose index"=w567) -> ("Boolean"=w572:bool)
                n268 = case shown="True" w572 {
                  tunnel: w571 -> [w574 w580]
                  tunnel: [w574 w579] -> w570
                  tunnel: w569 -> [w573 w578]
                  tunnel: [w573 w576] -> w568
                  tunnel: w567 -> [_ w577]
                  frame False {
                  }
                  frame True {
                    n269 = Build Array (concatenate)(w578, w577) -> (w576:i32[])
                    n270 = Decrement(x=w580) -> (x-1=w579:i32)
                    n271 = property on="Boolean 30" class="Bool"("DisabledEnum"=T2."Disabled and Grayed Out" ("Disabled")) -> ()  [unwired: 2 in, 2 out]
                  }
                }
              }
              frame 30 {
                n272 = call "select_seat_comfirm.vi"("choose index"=w581) -> ("Boolean"=w586:bool)
                n273 = case shown="True" w586 {
                  tunnel: w585 -> [w588 w594]
                  tunnel: [w588 w593] -> w584
                  tunnel: w583 -> [w587 w592]
                  tunnel: [w587 w590] -> w582
                  tunnel: w581 -> [_ w591]
                  frame False {
                  }
                  frame True {
                    n274 = Build Array (concatenate)(w592, w591) -> (w590:i32[])
                    n275 = Decrement(x=w594) -> (x-1=w593:i32)
                    n276 = property on="Boolean 31" class="Bool"("DisabledEnum"=T2."Disabled and Grayed Out" ("Disabled")) -> ()  [unwired: 2 in, 2 out]
                  }
                }
              }
              frame 31 {
                n277 = call "select_seat_comfirm.vi"("choose index"=w595) -> ("Boolean"=w600:bool)
                n278 = case shown="True" w600 {
                  tunnel: w599 -> [w602 w608]
                  tunnel: [w602 w607] -> w598
                  tunnel: w597 -> [w601 w606]
                  tunnel: [w601 w604] -> w596
                  tunnel: w595 -> [_ w605]
                  frame False {
                  }
                  frame True {
                    n279 = Build Array (concatenate)(w606, w605) -> (w604:i32[])
                    n280 = Decrement(x=w608) -> (x-1=w607:i32)
                    n281 = property on="Boolean 32" class="Bool"("DisabledEnum"=T2."Disabled and Grayed Out" ("Disabled")) -> ()  [unwired: 2 in, 2 out]
                  }
                }
              }
              frame 32 {
                n282 = call "select_seat_comfirm.vi"("choose index"=w609) -> ("Boolean"=w614:bool)
                n283 = case shown="True" w614 {
                  tunnel: w613 -> [w616 w622]
                  tunnel: [w616 w621] -> w612
                  tunnel: w611 -> [w615 w620]
                  tunnel: [w615 w618] -> w610
                  tunnel: w609 -> [_ w619]
                  frame False {
                  }
                  frame True {
                    n284 = Build Array (concatenate)(w620, w619) -> (w618:i32[])
                    n285 = Decrement(x=w622) -> (x-1=w621:i32)
                    n286 = property on="Boolean 33" class="Bool"("DisabledEnum"=T2."Disabled and Grayed Out" ("Disabled")) -> ()  [unwired: 2 in, 2 out]
                  }
                }
              }
              frame 33 {
                n287 = call "select_seat_comfirm.vi"("choose index"=w623) -> ("Boolean"=w628:bool)
                n288 = case shown="True" w628 {
                  tunnel: w627 -> [w630 w636]
                  tunnel: [w630 w635] -> w626
                  tunnel: w625 -> [w629 w634]
                  tunnel: [w629 w632] -> w624
                  tunnel: w623 -> [_ w633]
                  frame False {
                  }
                  frame True {
                    n289 = Build Array (concatenate)(w634, w633) -> (w632:i32[])
                    n290 = Decrement(x=w636) -> (x-1=w635:i32)
                    n291 = property on="Boolean 34" class="Bool"("DisabledEnum"=T2."Disabled and Grayed Out" ("Disabled")) -> ()  [unwired: 2 in, 2 out]
                  }
                }
              }
              frame 34 {
                n292 = call "select_seat_comfirm.vi"("choose index"=w637) -> ("Boolean"=w642:bool)
                n293 = case shown="True" w642 {
                  tunnel: w641 -> [w644 w650]
                  tunnel: [w644 w649] -> w640
                  tunnel: w639 -> [w643 w648]
                  tunnel: [w643 w646] -> w638
                  tunnel: w637 -> [_ w647]
                  frame False {
                  }
                  frame True {
                    n294 = Build Array (concatenate)(w648, w647) -> (w646:i32[])
                    n295 = Decrement(x=w650) -> (x-1=w649:i32)
                    n296 = property on="Boolean 35" class="Bool"("DisabledEnum"=T2."Disabled and Grayed Out" ("Disabled")) -> ()  [unwired: 2 in, 2 out]
                  }
                }
              }
              frame 35 {
                n297 = call "select_seat_comfirm.vi"("choose index"=w651) -> ("Boolean"=w656:bool)
                n298 = case shown="True" w656 {
                  tunnel: w655 -> [w658 w664]
                  tunnel: [w658 w663] -> w654
                  tunnel: w653 -> [w657 w662]
                  tunnel: [w657 w660] -> w652
                  tunnel: w651 -> [_ w661]
                  frame False {
                  }
                  frame True {
                    n299 = Build Array (concatenate)(w662, w661) -> (w660:i32[])
                    n300 = Decrement(x=w664) -> (x-1=w663:i32)
                    n301 = property on="Boolean 36" class="Bool"("DisabledEnum"=T2."Disabled and Grayed Out" ("Disabled")) -> ()  [unwired: 2 in, 2 out]
                  }
                }
              }
              frame 36 {
                n302 = call "select_seat_comfirm.vi"("choose index"=w665) -> ("Boolean"=w670:bool)
                n303 = case shown="True" w670 {
                  tunnel: w669 -> [w672 w678]
                  tunnel: [w672 w677] -> w668
                  tunnel: w667 -> [w671 w676]
                  tunnel: [w671 w674] -> w666
                  tunnel: w665 -> [_ w675]
                  frame False {
                  }
                  frame True {
                    n304 = Build Array (concatenate)(w676, w675) -> (w674:i32[])
                    n305 = Decrement(x=w678) -> (x-1=w677:i32)
                    n306 = property on="Boolean 37" class="Bool"("DisabledEnum"=T2."Disabled and Grayed Out" ("Disabled")) -> ()  [unwired: 2 in, 2 out]
                  }
                }
              }
              frame 37 {
                n307 = call "select_seat_comfirm.vi"("choose index"=w679) -> ("Boolean"=w684:bool)
                n308 = case shown="True" w684 {
                  tunnel: w683 -> [w686 w692]
                  tunnel: [w686 w691] -> w682
                  tunnel: w681 -> [w685 w690]
                  tunnel: [w685 w688] -> w680
                  tunnel: w679 -> [_ w689]
                  frame False {
                  }
                  frame True {
                    n309 = Build Array (concatenate)(w690, w689) -> (w688:i32[])
                    n310 = Decrement(x=w692) -> (x-1=w691:i32)
                    n311 = property on="Boolean 38" class="Bool"("DisabledEnum"=T2."Disabled and Grayed Out" ("Disabled")) -> ()  [unwired: 2 in, 2 out]
                  }
                }
              }
              frame 38 {
                n312 = call "select_seat_comfirm.vi"("choose index"=w693) -> ("Boolean"=w698:bool)
                n313 = case shown="True" w698 {
                  tunnel: w697 -> [w700 w706]
                  tunnel: [w700 w705] -> w696
                  tunnel: w695 -> [w699 w704]
                  tunnel: [w699 w702] -> w694
                  tunnel: w693 -> [_ w703]
                  frame False {
                  }
                  frame True {
                    n314 = Build Array (concatenate)(w704, w703) -> (w702:i32[])
                    n315 = Decrement(x=w706) -> (x-1=w705:i32)
                    n316 = property on="Boolean 39" class="Bool"("DisabledEnum"=T2."Disabled and Grayed Out" ("Disabled")) -> ()  [unwired: 2 in, 2 out]
                  }
                }
              }
              frame 39 {
                n317 = call "select_seat_comfirm.vi"("choose index"=w707) -> ("Boolean"=w712:bool)
                n318 = case shown="True" w712 {
                  tunnel: w711 -> [w714 w720]
                  tunnel: [w714 w719] -> w710
                  tunnel: w709 -> [w713 w718]
                  tunnel: [w713 w716] -> w708
                  tunnel: w707 -> [_ w717]
                  frame False {
                  }
                  frame True {
                    n319 = Build Array (concatenate)(w718, w717) -> (w716:i32[])
                    n320 = Decrement(x=w720) -> (x-1=w719:i32)
                    n321 = property on="Boolean 40" class="Bool"("DisabledEnum"=T2."Disabled and Grayed Out" ("Disabled")) -> ()  [unwired: 2 in, 2 out]
                  }
                }
              }
              frame 40 {
                n322 = call "select_seat_comfirm.vi"("choose index"=w721) -> ("Boolean"=w726:bool)
                n323 = case shown="True" w726 {
                  tunnel: w725 -> [w728 w734]
                  tunnel: [w728 w733] -> w724
                  tunnel: w723 -> [w727 w732]
                  tunnel: [w727 w730] -> w722
                  tunnel: w721 -> [_ w731]
                  frame False {
                  }
                  frame True {
                    n324 = Build Array (concatenate)(w732, w731) -> (w730:i32[])
                    n325 = Decrement(x=w734) -> (x-1=w733:i32)
                    n326 = property on="Boolean 41" class="Bool"("DisabledEnum"=T2."Disabled and Grayed Out" ("Disabled")) -> ()  [unwired: 2 in, 2 out]
                  }
                }
              }
              frame 41 {
                n327 = call "select_seat_comfirm.vi"("choose index"=w735) -> ("Boolean"=w740:bool)
                n328 = case shown="True" w740 {
                  tunnel: w739 -> [w742 w748]
                  tunnel: [w742 w747] -> w738
                  tunnel: w737 -> [w741 w746]
                  tunnel: [w741 w744] -> w736
                  tunnel: w735 -> [_ w745]
                  frame False {
                  }
                  frame True {
                    n329 = Build Array (concatenate)(w746, w745) -> (w744:i32[])
                    n330 = Decrement(x=w748) -> (x-1=w747:i32)
                    n331 = property on="Boolean 42" class="Bool"("DisabledEnum"=T2."Disabled and Grayed Out" ("Disabled")) -> ()  [unwired: 2 in, 2 out]
                  }
                }
              }
              frame 42 {
                n332 = call "select_seat_comfirm.vi"("choose index"=w749) -> ("Boolean"=w754:bool)
                n333 = case shown="True" w754 {
                  tunnel: w753 -> [w756 w762]
                  tunnel: [w756 w761] -> w752
                  tunnel: w751 -> [w755 w760]
                  tunnel: [w755 w758] -> w750
                  tunnel: w749 -> [_ w759]
                  frame False {
                  }
                  frame True {
                    n334 = Build Array (concatenate)(w760, w759) -> (w758:i32[])
                    n335 = Decrement(x=w762) -> (x-1=w761:i32)
                    n336 = property on="Boolean 43" class="Bool"("DisabledEnum"=T2."Disabled and Grayed Out" ("Disabled")) -> ()  [unwired: 2 in, 2 out]
                  }
                }
              }
              frame 43 {
                n337 = call "select_seat_comfirm.vi"("choose index"=w763) -> ("Boolean"=w768:bool)
                n338 = case shown="True" w768 {
                  tunnel: w767 -> [w770 w776]
                  tunnel: [w770 w775] -> w766
                  tunnel: w765 -> [w769 w774]
                  tunnel: [w769 w772] -> w764
                  tunnel: w763 -> [_ w773]
                  frame False {
                  }
                  frame True {
                    n339 = Build Array (concatenate)(w774, w773) -> (w772:i32[])
                    n340 = Decrement(x=w776) -> (x-1=w775:i32)
                    n341 = property on="Boolean 44" class="Bool"("DisabledEnum"=T2."Disabled and Grayed Out" ("Disabled")) -> ()  [unwired: 2 in, 2 out]
                  }
                }
              }
              frame 44 {
                n342 = call "select_seat_comfirm.vi"("choose index"=w777) -> ("Boolean"=w782:bool)
                n343 = case shown="True" w782 {
                  tunnel: w781 -> [w784 w790]
                  tunnel: [w784 w789] -> w780
                  tunnel: w779 -> [w783 w788]
                  tunnel: [w783 w786] -> w778
                  tunnel: w777 -> [_ w787]
                  frame False {
                  }
                  frame True {
                    n344 = Build Array (concatenate)(w788, w787) -> (w786:i32[])
                    n345 = Decrement(x=w790) -> (x-1=w789:i32)
                    n346 = property on="Boolean 45" class="Bool"("DisabledEnum"=T2."Disabled and Grayed Out" ("Disabled")) -> ()  [unwired: 2 in, 2 out]
                  }
                }
              }
              frame 45 {
                n347 = call "select_seat_comfirm.vi"("choose index"=w791) -> ("Boolean"=w796:bool)
                n348 = case shown="True" w796 {
                  tunnel: w795 -> [w798 w804]
                  tunnel: [w798 w803] -> w794
                  tunnel: w793 -> [w797 w802]
                  tunnel: [w797 w800] -> w792
                  tunnel: w791 -> [_ w801]
                  frame False {
                  }
                  frame True {
                    n349 = Build Array (concatenate)(w802, w801) -> (w800:i32[])
                    n350 = Decrement(x=w804) -> (x-1=w803:i32)
                    n351 = property on="Boolean 46" class="Bool"("DisabledEnum"=T2."Disabled and Grayed Out" ("Disabled")) -> ()  [unwired: 2 in, 2 out]
                  }
                }
              }
              frame 46 {
                n352 = call "select_seat_comfirm.vi"("choose index"=w805) -> ("Boolean"=w810:bool)
                n353 = case shown="True" w810 {
                  tunnel: w809 -> [w812 w818]
                  tunnel: [w812 w817] -> w808
                  tunnel: w807 -> [w811 w816]
                  tunnel: [w811 w814] -> w806
                  tunnel: w805 -> [_ w815]
                  frame False {
                  }
                  frame True {
                    n354 = Build Array (concatenate)(w816, w815) -> (w814:i32[])
                    n355 = Decrement(x=w818) -> (x-1=w817:i32)
                    n356 = property on="Boolean 47" class="Bool"("DisabledEnum"=T2."Disabled and Grayed Out" ("Disabled")) -> ()  [unwired: 2 in, 2 out]
                  }
                }
              }
              frame 47 {
                n357 = call "select_seat_comfirm.vi"("choose index"=w819) -> ("Boolean"=w824:bool)
                n358 = case shown="True" w824 {
                  tunnel: w823 -> [w826 w832]
                  tunnel: [w826 w831] -> w822
                  tunnel: w821 -> [w825 w830]
                  tunnel: [w825 w828] -> w820
                  tunnel: w819 -> [_ w829]
                  frame False {
                  }
                  frame True {
                    n359 = Build Array (concatenate)(w830, w829) -> (w828:i32[])
                    n360 = Decrement(x=w832) -> (x-1=w831:i32)
                    n361 = property on="Boolean 48" class="Bool"("DisabledEnum"=T2."Disabled and Grayed Out" ("Disabled")) -> ()  [unwired: 2 in, 2 out]
                  }
                }
              }
              frame 48, Default {
              }
            }
            n362 = Increment(x=w147) -> (x+1=w148:i32)
            n363 = Subtract(x=w148, y=w151) -> (x-y=→"th seat you choose":i32)
            n364 = Less Or Equal To 0?(x=w151) -> (x <= 0?=w153:bool)
            n365 = Or(x=w153, y="stop") -> (x .or. y?=w154:bool)
          }
          n366 = case shown="False" w134 {
            tunnel: [w143 w146] -> w138
            tunnel: w137 -> [w141 _]
            tunnel: w136 -> [w142 w146]
            tunnel: [w141 i32[] [] ("Array")] -> w135
            tunnel: [w140 0 ("No. of seats want to choose")] -> w132
            tunnel: w131 -> [w140 _]
            frame False {
              n367 = Build Array (concatenate)(w142, w141) -> (w143:i32[])
            }
            frame True {
            }
          }
        }
        frame True {
          w836 = i32[] [] ("Array")
        }
      }
    }
  }
  "Cancel" <- w4
  "No. of seats choosen" <- w3
  n368 = Sort 1D Array(array=w6) -> (sorted array=→"selected seats after":i32[])
  n369 = Sort 1D Array(array=w7) -> (sorted array=→"seats selected by user":i32[])
